vi "Get Existing File.vi"(7 "action if file doesn't exist (0: prompt for existing)":T1, 8 "error in (no error)":errorcluster, 11 "file path in":path) -> (0 "error out":errorcluster, 3 "file path out":path)   [LabVIEW 2018, in "ASI TG-1000.lvlib"]
doc: "Queries the ASI controller for the position along the specified axes and saves the result to a file for later use."
uses:
  ASI TG-1000.lvlib
  File action if doesn't exist.ctl
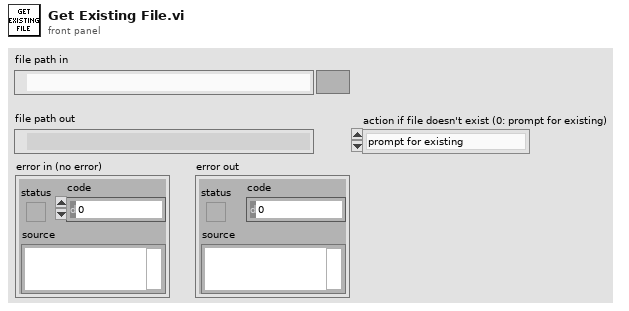
[diagram p1: front panel]
types:
  T1 = typedef "ASI TG-1000.lvlib/File action if doesn't exist.ctl" = enum16{"prompt for existing", "try to create, prompt if can't", "try to create, error if can't"}
  T2 = enum16{"open", "replace", "create", "open or create", "replace or create", "replace or create with confirmation"}
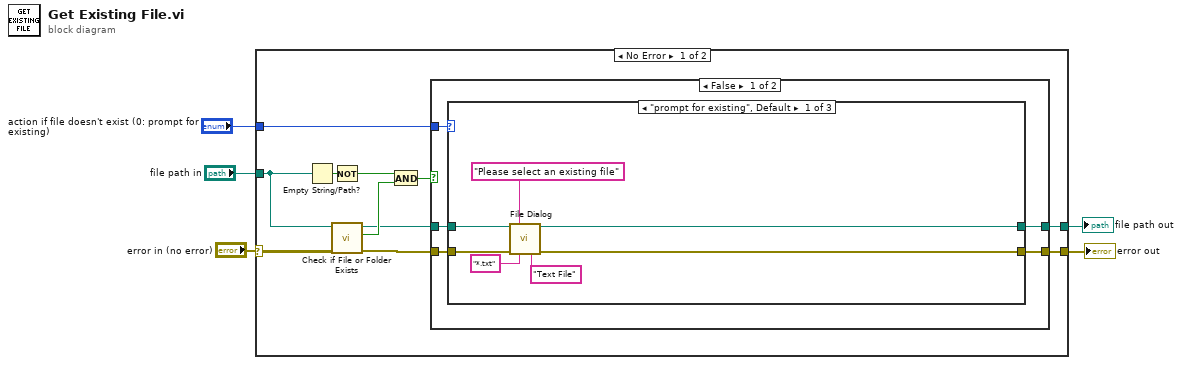
[diagram p0: block diagram]
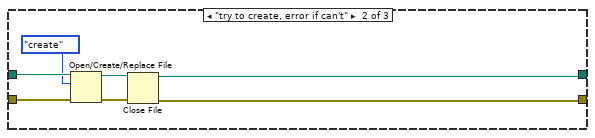
[diagram p2: hidden frame]
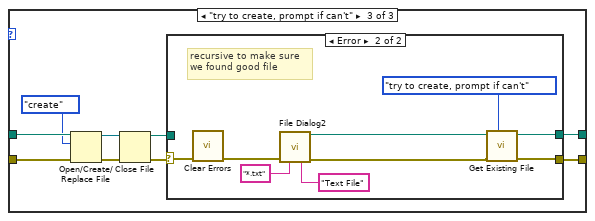
[diagram p3: hidden frame]
diagram:
  n1 = case shown="No Error" "error in (no error)" {
    selector: "error in (no error)" -> [w16 w59]
    tunnel: [w7 w59] -> w5
    tunnel: "file path in" -> [w12 w58]
    tunnel: [w9 w58] -> w2
    tunnel: "action if file doesn't exist (0: prompt for existing)" -> [w6 _]
    frame No Error {
      n2 = Empty String/Path?(string/path=w12) -> (empty?=w15:bool)
      n3 = Not(x=w15) -> (.not. x?=w14:bool)
      n4 = call <vilib>:"Check if File or Folder Exists.vi"("error in (no error)"=w16, "path"=w12) -> ("error out"=w8:errorcluster, "file or folder exists?"=w13:bool, "dup path"=w10:path)  [unwired: 7 in]
      n5 = And(x=w14, y=w13) -> (x .and. y?=w11:bool)
      n6 = case shown="False" w11 {
        tunnel: w10 -> [w19 w57]
        tunnel: [w18 w57] -> w9
        tunnel: w8 -> [w21 w56]
        tunnel: [w20 w56] -> w7
        tunnel: w6 -> [w17 _]
        frame False {
          n7 = case shown="\"prompt for existing\", Default" w17 {
            tunnel: w21 -> [w28 w35 w44]
            tunnel: [w24 w30 w40] -> w20
            tunnel: w19 -> [w27 w34 w43]
            tunnel: [w23 w29 w41] -> w18
            frame "prompt for existing", Default {
              n8 = call "File Dialog"("start path"=w27, "prompt"="Please select an existing file", "error in"=w28, "pattern (all files)"="*.txt", "pattern label"="Text File") -> ("selected path"=w23:path, "error out"=w24:errorcluster)  [unwired: 7 in, 2 out]
            }
            frame "try to create, error if can't" {
              n9 = Open/Create/Replace File(file path (use dialog)=w34, error in=w35, operation (0:open)=T2."create") -> (refnum out=w31:refnum<file>, error out=w32:errorcluster)  [unwired: 3 in, 1 out]
              n10 = Close File(refnum=w31, error in=w32) -> (path=w29:path, error out=w30:errorcluster)
            }
            frame "try to create, prompt if can't" {
              n11 = Open/Create/Replace File(file path (use dialog)=w43, error in=w44, operation (0:open)=T2."create") -> (refnum out=w38:refnum<file>, error out=w39:errorcluster)  [unwired: 3 in, 1 out]
              n12 = Close File(refnum=w38, error in=w39) -> (path=w36:path, error out=w37:errorcluster)
              n13 = case shown="Error" w37 {
                selector: w37 -> [w46 w53]
                tunnel: [w45 w51] -> w41
                tunnel: [w46 w50] -> w40
                tunnel: w36 -> [w45 _]
                frame No Error {
                }
                frame Error {
                  # "recursive to make sure \nwe found good file"
                  n14 = call <vilib>:"Clear Errors.vi"("error in (no error)"=w53) -> ("error out"=w52:errorcluster)  [unwired: 5 in, 1 out]
                  n15 = call "File Dialog2"("error in"=w52, "pattern (all files)"="*.txt", "pattern label"="Text File") -> ("selected path"=w48:path, "error out"=w47:errorcluster)  [unwired: 9 in, 2 out]
                  n16 = call "Get Existing File.vi"("action if file doesn't exist (0: prompt for existing)"=File_action_if_doesn't_exist."try to create, prompt if can't" ("action if doesn't exist"), "error in (no error)"=w47, "file path in"=w48) -> ("error out"=w50:errorcluster, "file path out"=w51:path)  [unwired: 7 in]
                }
              }
            }
          }
        }
        frame True {
        }
      }
    }
    frame Error {
    }
  }
  "error out" <- w5
  "file path out" <- w2
